vi "which laser.vi"(11 "Laser Data":dbl[][](array[numeric])) -> (3 "WhichLaser":i32[](array[numeric]))   [LabVIEW 2015]
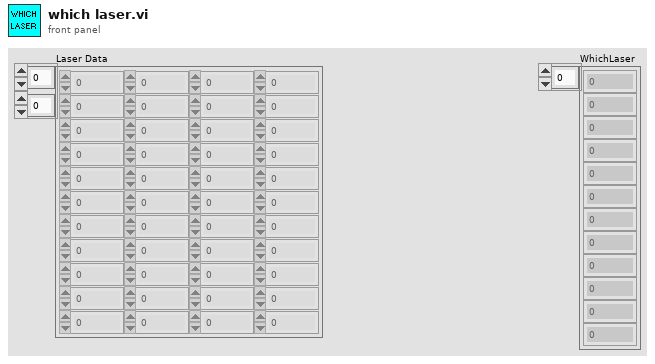
[diagram p1: front panel]
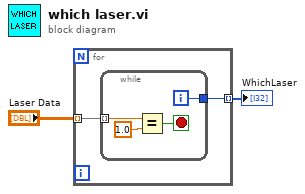
[diagram p0: block diagram]
diagram:
  n1 = for {
    tunnel: "Laser Data" -> [w4] mode=indexing
    tunnel: [w3] -> w1 mode=indexing
    n2 = while {
      tunnel: w4 -> [w7] mode=indexing
      tunnel: [w5] -> w3
      i -> [w5]
      stop <- w6 stop-if-true
      n3 = Equal?(x=w7, y=1.0) -> (x = y?=w6:bool)
    }
  }
  "WhichLaser" <- w1
